vi "2 Global.vi"() -> ()   [LabVIEW 2011]
uses:
  2 Typedefs/UTM Location.ctl
  2 Typedefs/apparent wind.ctl
  2 Typedefs/apparent wind speed.ctl
  2 Typedefs/apparent wind direction.ctl
  2 Typedefs/Velocity.ctl
  2 Typedefs/heading.ctl
  2 Typedefs/generalized actuator status.ctl
  2 Typedefs/indicator LED.ctl
  2 Typedefs/generalized sensor status.ctl
  2 Typedefs/manual override.ctl
  2 Typedefs/setpoints to boat.ctl
  2 Typedefs/sail setpt.ctl
  2 Typedefs/rudder angle.ctl
panel:
  in  "Globals":T1(tab)
  in  "Which Boat Am I?":u16(ring) items=["Small RC", "Large RC", "Final Boat", "Simulator"]
  out "Direction Sensor Status":T2
  out "Location Sensor Status":T2
  out "Wind Sensor Status":T2
  out "Sail Actuator Status":T4
  out "Rudder Actuator Status":T4
  in  "Battery Voltage":dbl
  in  "Robot\nHeading":T5 format="%05.1f"
  in  "Robot UTM Location":T6
  in  "Robot Velocity":T7
  in  "Absolute Wind":T7
  in  "Apparent Wind\nDirection":T8
  in  "Apparent Wind\nSpeed":T9
  in  "Apparent Wind":T10
  in  "Setpoints to boat":T11
  in  "Manual Override Cluster":T14
  in  "Sail Position":T12
  in  "Rudder Angle":T13
  # "All distances in meters, all speeds in meters per second\nAll angles in degrees, clockwise with 0 being positive North if in global reference frame or 0 being Fore in boat ref frame.\nX-Y make a right handed coordinate system with Z pointing up\nPositive Rudder angle makes the boat turn right\nLocation Coordinates are in UTM format"
  # "As Measured"
  # "From Planning Functions"
  # "Path Planning"
  # "(this is not a cluster because subitems\nare generated in parallel code)"
  # "Mission Definition Stuff Goes HERE"
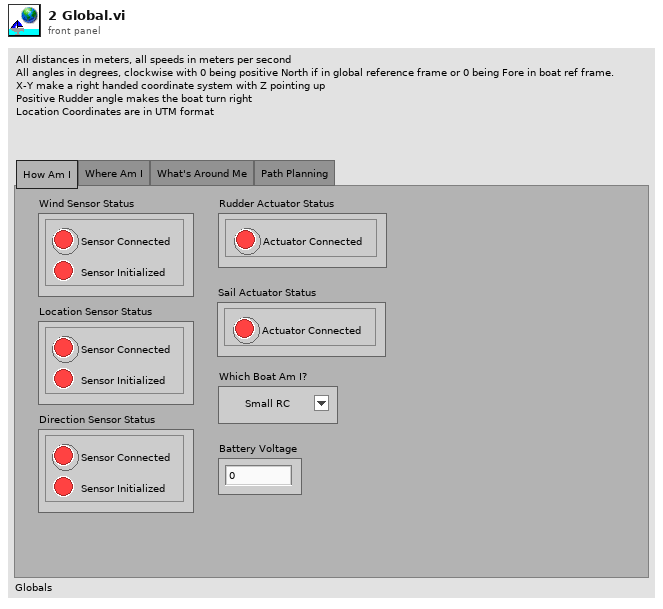
[diagram p1: front panel]
types:
  T1 = enum32{"How Am I", "Where Am I", "What's Around Me", "Path Planning"}
  T2 = typedef "generalized sensor status.ctl" = cluster{"Sensor Connected":T3, "Sensor Initialized":T3}
  T3 = typedef "indicator LED.ctl" = bool
  T4 = typedef "generalized actuator status.ctl" = cluster{"Actuator Connected":T3}
  T5 = typedef "heading.ctl" = dbl
  T6 = typedef "UTM Location.ctl" = cluster{"UTM Zone":dbl, "Hemisphere":enum16{"North", "South"}, "East":dbl, "North":dbl}
  T7 = typedef "Velocity.ctl" = cluster{"East":dbl, "North":dbl}
  T8 = typedef "apparent wind direction.ctl" = dbl
  T9 = typedef "apparent wind speed.ctl" = dbl
  T10 = typedef "apparent wind.ctl" = cluster{"Toward Fore":dbl, "Toward Starboard":dbl}
  T11 = typedef "setpoints to boat.ctl" = cluster{"Sail Position":T12, "Rudder Angle":T13}
  T12 = typedef "sail setpt.ctl" = dbl
  T13 = typedef "rudder angle.ctl" = dbl
  T14 = typedef "manual override.ctl" = cluster{"Override Active":bool, "Setpoints":T11}
diagram:
